vi "mySweepSelect.vi"(0 "实际使用的注入模式":u8(ring) items=["单相", "三相αβ系", "三相同步系", "三相正负序"], 1 "f_tick_min":u32=1, 2 "f_mes_max":u32=5000, 5 "freqs, measu. coups":i32[][](array[numeric]), 7 "freqs groups":i32[][][](array[numeric]), 9 "index group":i32[][](array[numeric]), 11 "ix":i32, 12 "同步频率上限 f_tick_ref":u32, 13 "测量周期数 n":u32=2 min=1 max=10) -> (3 "f_tick":dbl, 4 "注入小模式":u8, 6 "freq rows":i32[][](array[numeric]), 8 "index row":i32[](array[numeric]), 10 "sample":u64=127, 14 "f_mes":i32, 15 "timebase":u32=127)   [LabVIEW 2024]
doc: "在扫频循环内，注入模式（允许100）被进一步细分为小注入模式。\n小模式：0 - 稳态，仅测量\n1 - 单相注入\n2 - 三相α注入\n3 - 三相β注入\n4 - 三相d注入\n5 - 三相q注入\n6 - 三相正负序注入\n100 - 能注就注，能测就测，不计算响应"
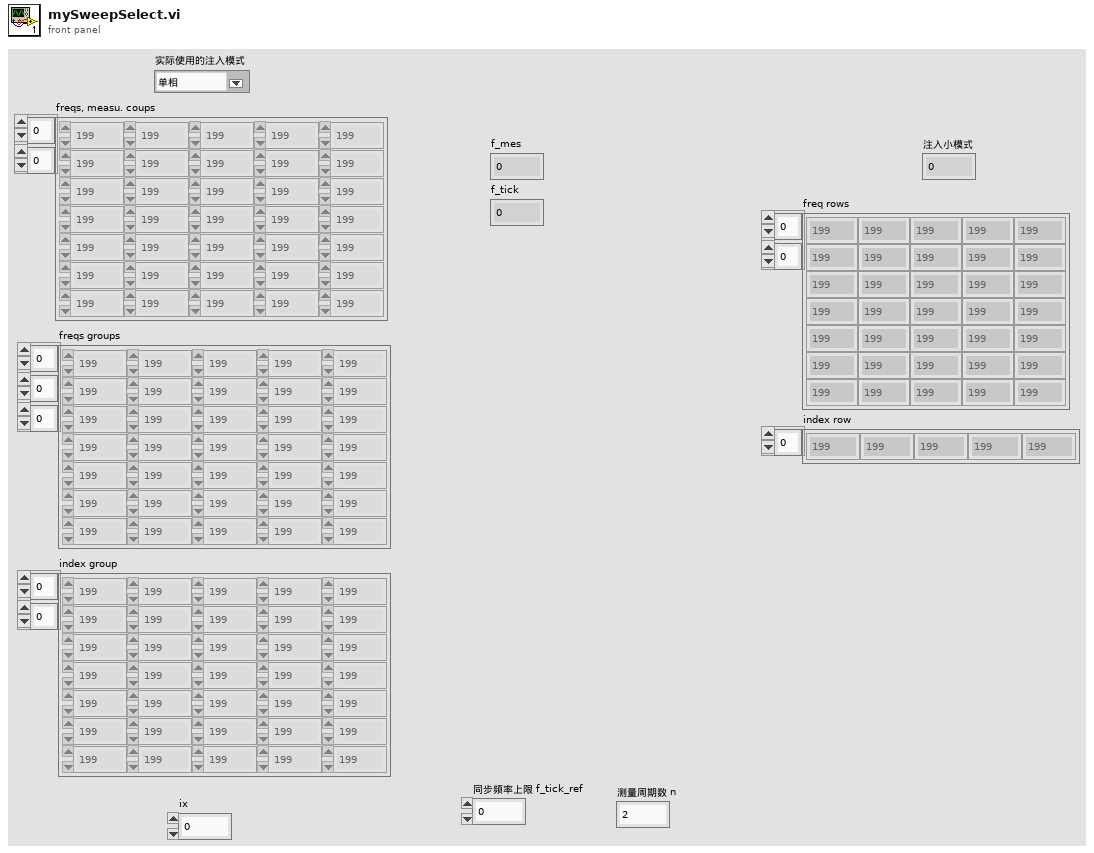
[diagram p1: front panel]
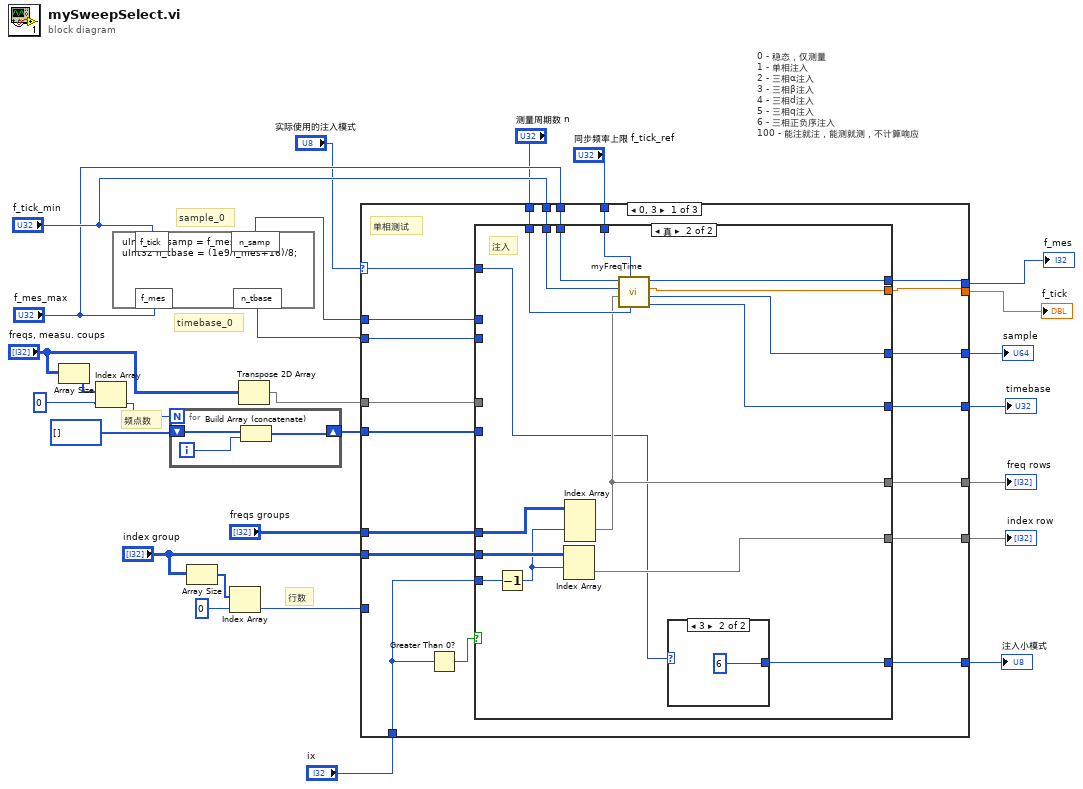
[diagram p0: block diagram]
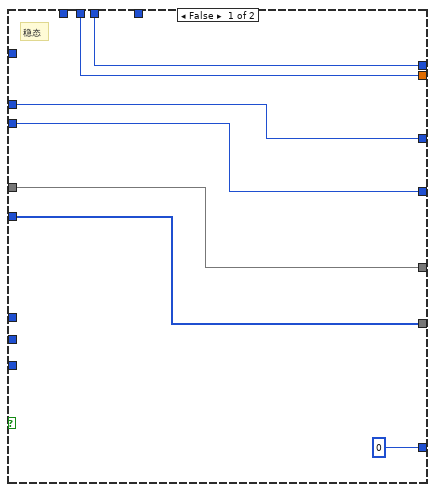
[diagram p2: hidden frame]
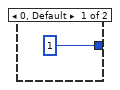
[diagram p3: hidden frame]
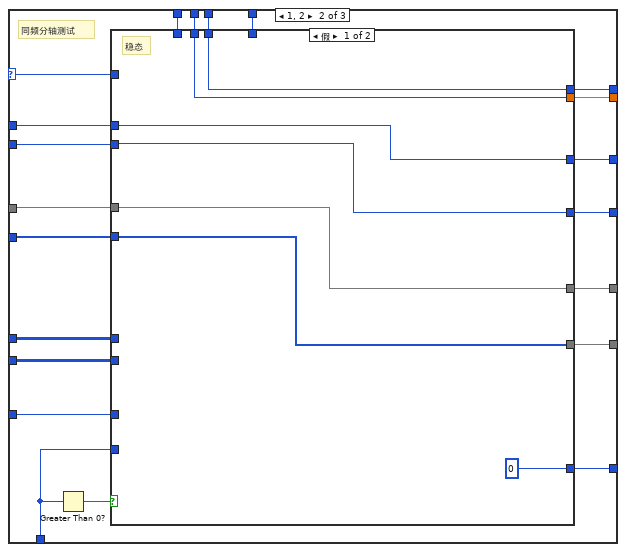
[diagram p4: hidden frame]
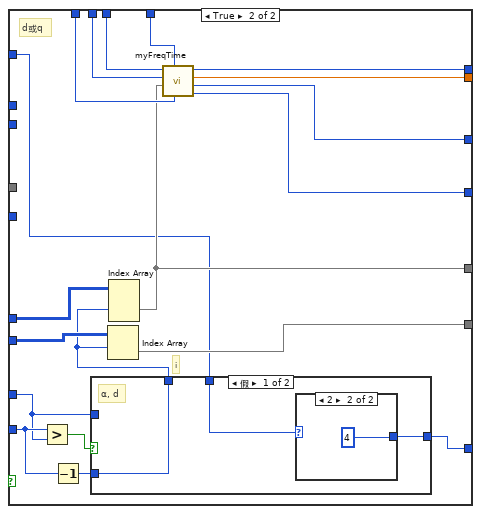
[diagram p5: hidden frame]
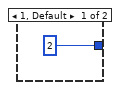
[diagram p6: hidden frame]
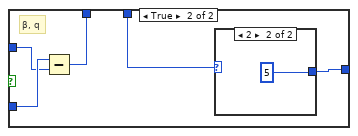
[diagram p7: hidden frame]
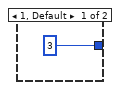
[diagram p8: hidden frame]
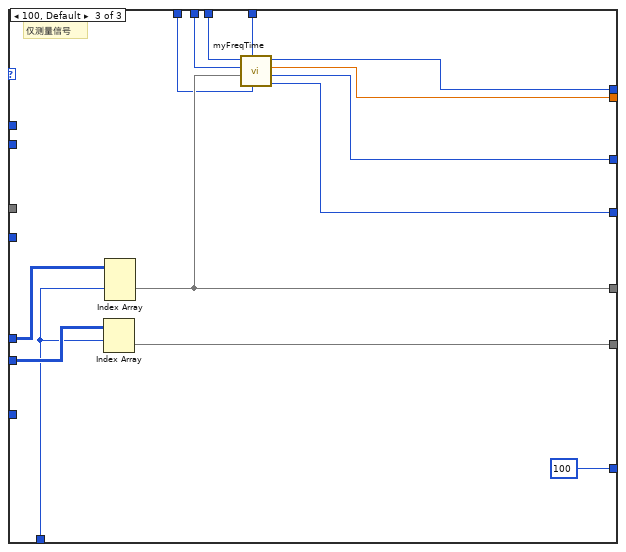
[diagram p9: hidden frame]
diagram:
  # "0 - 稳态，仅测量\n1 - 单相注入\n2 - 三相α注入\n3 - 三相β注入\n4 - 三相d注入\n5 - 三相q注入\n6 - 三相正负序注入\n100 - 能注就注，能测就测，不计算响应"
  # "频点数"
  # "行数"
  # "timebase_0"
  # "sample_0"
  n1 = Array Size(array="freqs, measu. coups") -> (size(s)=w4:i32[])
  n2 = Index Array(array=w4, index=0 ("索引")) -> (element=w3:i32)
  n3 = formula code="uInt32 n_samp = f_mes/f_tick;\nuInt32 n_tbase = (1e9/f_mes+16)/8;"("f_tick"="f_tick_min", "f_mes"="f_mes_max") -> ("n_samp"=w24:u32, "n_tbase"=w25:u32)
  n4 = for {
    N: w3 -> [_]
    shift-right: [w28] -> w13
    shift-left: i32[] [] -> [w30]
    i -> [w29]
    n5 = Build Array (concatenate)(w30, w29) -> (w28:i32[])
  }
  n6 = Array Size(array="index group") -> (size(s)=w11:i32[])
  n7 = Index Array(array=w11, index=0 ("索引")) -> (element=w8:i32)
  n8 = Transpose 2D Array(2D array="freqs, measu. coups") -> (transposed array=w7:i32[][])
  n9 = case shown="0, 3" "实际使用的注入模式" {
    selector: "实际使用的注入模式" -> [w33 w78 _]
    tunnel: "ix" -> [w34 w91 w145]
    tunnel: "freqs groups" -> [w42 w84 w147]
    tunnel: [w50 w96 u8 100] -> w26
    tunnel: w24 -> [w49 w95 _]
    tunnel: w25 -> [w48 w94 _]
    tunnel: "index group" -> [w43 w83 w146]
    tunnel: "f_tick_min" -> [w39 w81 w142]
    tunnel: "f_mes_max" -> [w40 w80 w143]
    tunnel: [w45 w86 w141] -> w20
    tunnel: [w44 w85 w144] -> w19
    tunnel: "测量周期数 n" -> [w38 w82 w140]
    tunnel: "同步频率上限 f_tick_ref" -> [w41 w79 w139]
    tunnel: [w47 w88 w138] -> w16
    tunnel: [w46 w87 w137] -> w15
    tunnel: w7 -> [w37 w90 _]
    tunnel: w13 -> [w36 w89 _]
    tunnel: w8 -> [_ w93 _]
    tunnel: [w32 w77 w136] -> w2
    tunnel: [w31 w76 w135] -> w1
    frame 0, 3 {
      # "单相测试"
      n10 = Greater Than 0?(x=w34) -> (x > 0?=w35:bool)
      n11 = case shown="真" w35 {
        tunnel: [u8 0 w60] -> w50
        tunnel: w49 -> [w56 _]
        tunnel: w48 -> [w55 _]
        tunnel: [w56 w65] -> w47
        tunnel: [w55 w64] -> w46
        tunnel: [w53 w66] -> w45
        tunnel: [w54 w71] -> w44
        tunnel: w34 -> [_ w63]
        tunnel: w43 -> [_ w73]
        tunnel: w42 -> [_ w72]
        tunnel: w41 -> [_ w70]
        tunnel: w40 -> [w52 w69]
        tunnel: w39 -> [w51 w68]
        tunnel: w38 -> [_ w67]
        tunnel: w37 -> [w53 _]
        tunnel: w36 -> [w54 _]
        tunnel: w33 -> [_ w61]
        tunnel: [w52 w59] -> w32
        tunnel: [w51 w58] -> w31
        frame False {
          # "稳态"
        }
        frame True {
          # "注入"
          n12 = Decrement(x=w63) -> (x-1=w62:i32)
          n13 = Index Array(array=w73, index (row)=w62) -> (element=w71:i32[])  [unwired: 1 in]
          n14 = Index Array(array=w72, index (dim 1)=w62) -> (element=w66:i32[][])  [unwired: 2 in]
          n15 = call "myFreqTime.vi"("测量周期数 n"=w67, "同步频率上限 f_tick_ref"=w70, "freqs rows"=w66, "f_tick_min"=w68, "f_mes_max"=w69) -> ("n_tbase"=w64:u32, "n_samp"=w65:u64, "f_tick"=w58:dbl, "f_mes"=w59:i32)  [unwired: 1 in, 2 out]
          n16 = case shown="3" w61 {
            tunnel: [u8 1 u8 6] -> w60
            frame 0, Default {
            }
            frame 3 {
            }
          }
        }
      }
    }
    frame 1, 2 {
      # "同频分轴测试"
      n17 = Greater Than 0?(x=w91) -> (x > 0?=w92:bool)
      n18 = case shown="假" w92 {
        tunnel: [u8 0 w106] -> w96
        tunnel: w93 -> [_ w109]
        tunnel: w95 -> [w103 _]
        tunnel: w94 -> [w102 _]
        tunnel: w91 -> [_ w111]
        tunnel: w90 -> [w99 _]
        tunnel: w89 -> [w101 _]
        tunnel: [w103 w115] -> w88
        tunnel: [w102 w114] -> w87
        tunnel: [w99 w113] -> w86
        tunnel: [w101 w112] -> w85
        tunnel: w84 -> [_ w121]
        tunnel: w83 -> [_ w120]
        tunnel: w82 -> [_ w119]
        tunnel: w81 -> [w97 w118]
        tunnel: w80 -> [w98 w117]
        tunnel: w79 -> [_ w116]
        tunnel: w78 -> [_ w107]
        tunnel: [w98 w105] -> w77
        tunnel: [w97 w104] -> w76
        frame False {
          # "稳态"
        }
        frame True {
          # "i"
          # "d或q"
          n19 = Greater?(x=w111, y=w109) -> (0:w122:bool)
          n20 = Decrement(x=w111) -> (x-1=w110:i32)
          n21 = case shown="假" w122 {
            tunnel: w110 -> [w125 w132]
            tunnel: w109 -> [_ w131]
            tunnel: [w125 w130] -> w108
            tunnel: w107 -> [w123 w129]
            tunnel: [w124 w128] -> w106
            frame False {
              # "α, d"
              n22 = case shown="2" w123 {
                tunnel: [u8 2 u8 4] -> w124
                frame 1, Default {
                }
                frame 2 {
                }
              }
            }
            frame True {
              # "β, q"
              n23 = Subtract(x=w132, y=w131) -> (x-y=w130:i32)
              n24 = case shown="2" w129 {
                tunnel: [u8 3 u8 5] -> w128
                frame 1, Default {
                }
                frame 2 {
                }
              }
            }
          }
          n25 = Index Array(array=w120, index (row)=w108) -> (element=w112:i32[])  [unwired: 1 in]
          n26 = Index Array(array=w121, index (dim 1)=w108) -> (element=w113:i32[][])  [unwired: 2 in]
          n27 = call "myFreqTime.vi"("测量周期数 n"=w119, "同步频率上限 f_tick_ref"=w116, "freqs rows"=w113, "f_tick_min"=w118, "f_mes_max"=w117) -> ("n_tbase"=w114:u32, "n_samp"=w115:u64, "f_tick"=w104:dbl, "f_mes"=w105:i32)  [unwired: 1 in, 2 out]
        }
      }
    }
    frame 100, Default {
      # "仅测量信号"
      n28 = Index Array(array=w146, index (row)=w145) -> (element=w144:i32[])  [unwired: 1 in]
      n29 = Index Array(array=w147, index (dim 1)=w145) -> (element=w141:i32[][])  [unwired: 2 in]
      n30 = call "myFreqTime.vi"("测量周期数 n"=w140, "同步频率上限 f_tick_ref"=w139, "freqs rows"=w141, "f_tick_min"=w142, "f_mes_max"=w143) -> ("n_tbase"=w137:u32, "n_samp"=w138:u64, "f_tick"=w135:dbl, "f_mes"=w136:i32)  [unwired: 1 in, 2 out]
    }
  }
  "注入小模式" <- w26
  "sample" <- w16
  "timebase" <- w15
  "freq rows" <- w20
  "index row" <- w19
  "f_mes" <- w2
  "f_tick" <- w1
